vi "Read_INI.vi"(8 "error in (no error)":errorcluster, 11 "App_directory":path) -> (0 "error out":errorcluster, 2 "Options":T1={"Form_data_log_period"=0, "startup_threshold"=0.0, "Coeff_U"=2.55, "Offset_U"=6.5, "Coeff_I"=42.391, "Offset_I"=77.0, "Save_data_path"=path "", "ADC_frequency"=50000.0, "VISA resource name"="COM1"}, 3 "file path":path)   [LabVIEW 2012]
uses:
  Controls/options.ctl
  <vilib>/Utility/config.llb/Read Key (I32).vi
  <vilib>/Utility/config.llb/Read Key (Double).vi
  <vilib>/Utility/config.llb/Read Key (Path).vi
  <vilib>/Utility/config.llb/Read Key (String).vi
  <vilib>/Utility/config.llb/NI_LVConfig.lvlib
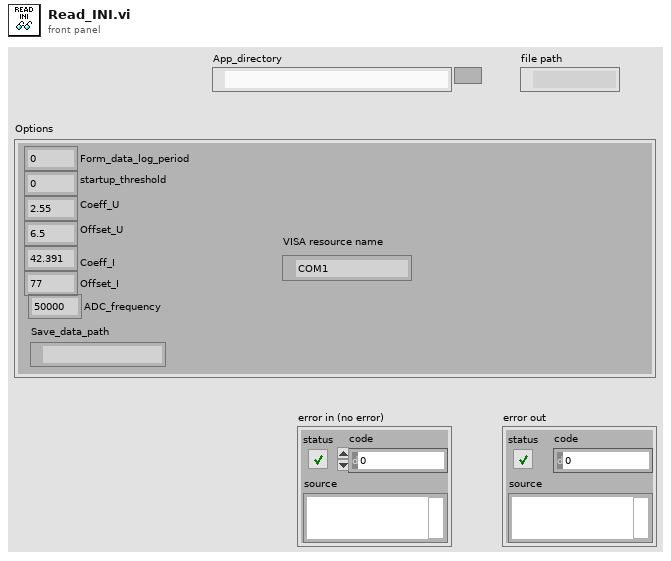
[diagram p1: front panel]
types:
  T1 = typedef "options.ctl" = cluster{"Form_data_log_period":i32, "startup_threshold":dbl, "Coeff_U":dbl, "Offset_U":dbl, "Coeff_I":dbl, "Offset_I":dbl, "Save_data_path":path, "ADC_frequency":dbl, "VISA resource name":refnum<visa-resource-name>}
  T2 = typedef "NI_LVConfig.lvlib/Config Data RefNum.ctl" = refnum<k1>
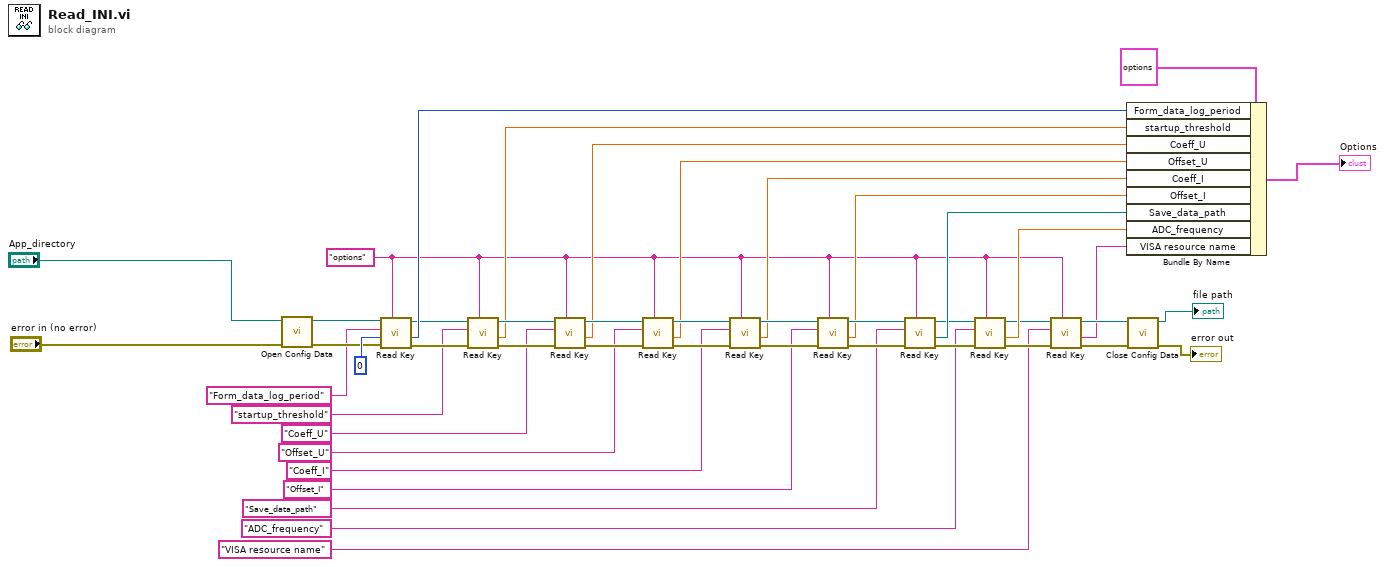
[diagram p0: block diagram]
diagram:
  w4 = "options" ("section")
  n1 = call <vilib>:"Open Config Data.vi"("error in (no error)"="error in (no error)", "configuration file path"="App_directory") -> ("error out"=w42:errorcluster, "refnum"=w41:T2)  [unwired: 7 in, 1 out]
  n2 = call-poly <vilib>:"Read Key.vi"("section"=w4, "error in (no error)"=w42, "default value"=0, "key"="Form_data_log_period", "refnum"=w41) -> ("error out"=w36:errorcluster, "value"=w39:i32, "refnum out"=w30:T2)  [unwired: 3 in, 1 out]
  n3 = call-poly <vilib>:"Read Key.vi"("section"=w4, "error in (no error)"=w36, "key"="startup_threshold", "refnum"=w30) -> ("error out"=w35:errorcluster, "value"=w18:dbl, "refnum out"=w29:T2)  [unwired: 4 in, 1 out]
  n4 = call-poly <vilib>:"Read Key.vi"("section"=w4, "error in (no error)"=w35, "key"="Coeff_U", "refnum"=w29) -> ("error out"=w34:errorcluster, "value"=w17:dbl, "refnum out"=w28:T2)  [unwired: 4 in, 1 out]
  n5 = call-poly <vilib>:"Read Key.vi"("section"=w4, "error in (no error)"=w34, "key"="Offset_U", "refnum"=w28) -> ("error out"=w33:errorcluster, "value"=w16:dbl, "refnum out"=w27:T2)  [unwired: 4 in, 1 out]
  n6 = call-poly <vilib>:"Read Key.vi"("section"=w4, "error in (no error)"=w33, "key"="Coeff_I", "refnum"=w27) -> ("error out"=w32:errorcluster, "value"=w15:dbl, "refnum out"=w26:T2)  [unwired: 4 in, 1 out]
  n7 = call-poly <vilib>:"Read Key.vi"("section"=w4, "error in (no error)"=w32, "key"="Offset_I", "refnum"=w26) -> ("error out"=w31:errorcluster, "value"=w14:dbl, "refnum out"=w25:T2)  [unwired: 4 in, 1 out]
  n8 = call-poly <vilib>:"Read Key.vi"("section"=w4, "error in (no error)"=w31, "key"="Save_data_path", "refnum"=w25) -> ("error out"=w11:errorcluster, "value"=w13:path, "refnum out"=w12:T2)  [unwired: 4 in, 1 out]
  n9 = call-poly <vilib>:"Read Key.vi"("section"=w4, "error in (no error)"=w11, "key"="ADC_frequency", "refnum"=w12) -> ("error out"=w6:errorcluster, "value"=w9:dbl, "refnum out"=w8:T2)  [unwired: 4 in, 1 out]
  n10 = call-poly <vilib>:"Read Key.vi"("section"=w4, "error in (no error)"=w6, "key"="VISA resource name", "refnum"=w8) -> ("error out"=w5:errorcluster, "value"=w2:string, "refnum out"=w7:T2)  [unwired: 4 in, 1 out]
  n11 = Bundle By Name(cluster=T1 {"Form_data_log_period"=0, "startup_threshold"=0.0, "Coeff_U"=0.0, "Offset_U"=0.0, "Coeff_I"=0.0, "Offset_I"=0.0, "Save_data_path"=path "", "ADC_frequency"=0.0, "VISA resource name"=""} ("Options"), "Form_data_log_period"=w39, "startup_threshold"=w18, "Coeff_U"=w17, "Offset_U"=w16, "Coeff_I"=w15, "Offset_I"=w14, "Save_data_path"=w13, "ADC_frequency"=w9, "VISA resource name"=w2) -> (→"Options":T1)
  n12 = call <vilib>:"Close Config Data.vi"("error in (no error)"=w5, "refnum"=w7) -> ("error out"=→"error out":errorcluster, "file path"=→"file path":path)  [unwired: 8 in]
